vi "AnalysisData2.vi"() -> ()   [LabVIEW 2011]
panel:
  out "RunningIndexStart 2":dbl
  out "RunningIndexStart":dbl
  out "子数组":string[](array[string])
  out "EXCEL读取":string[][](array[string])
  in  "路径":path
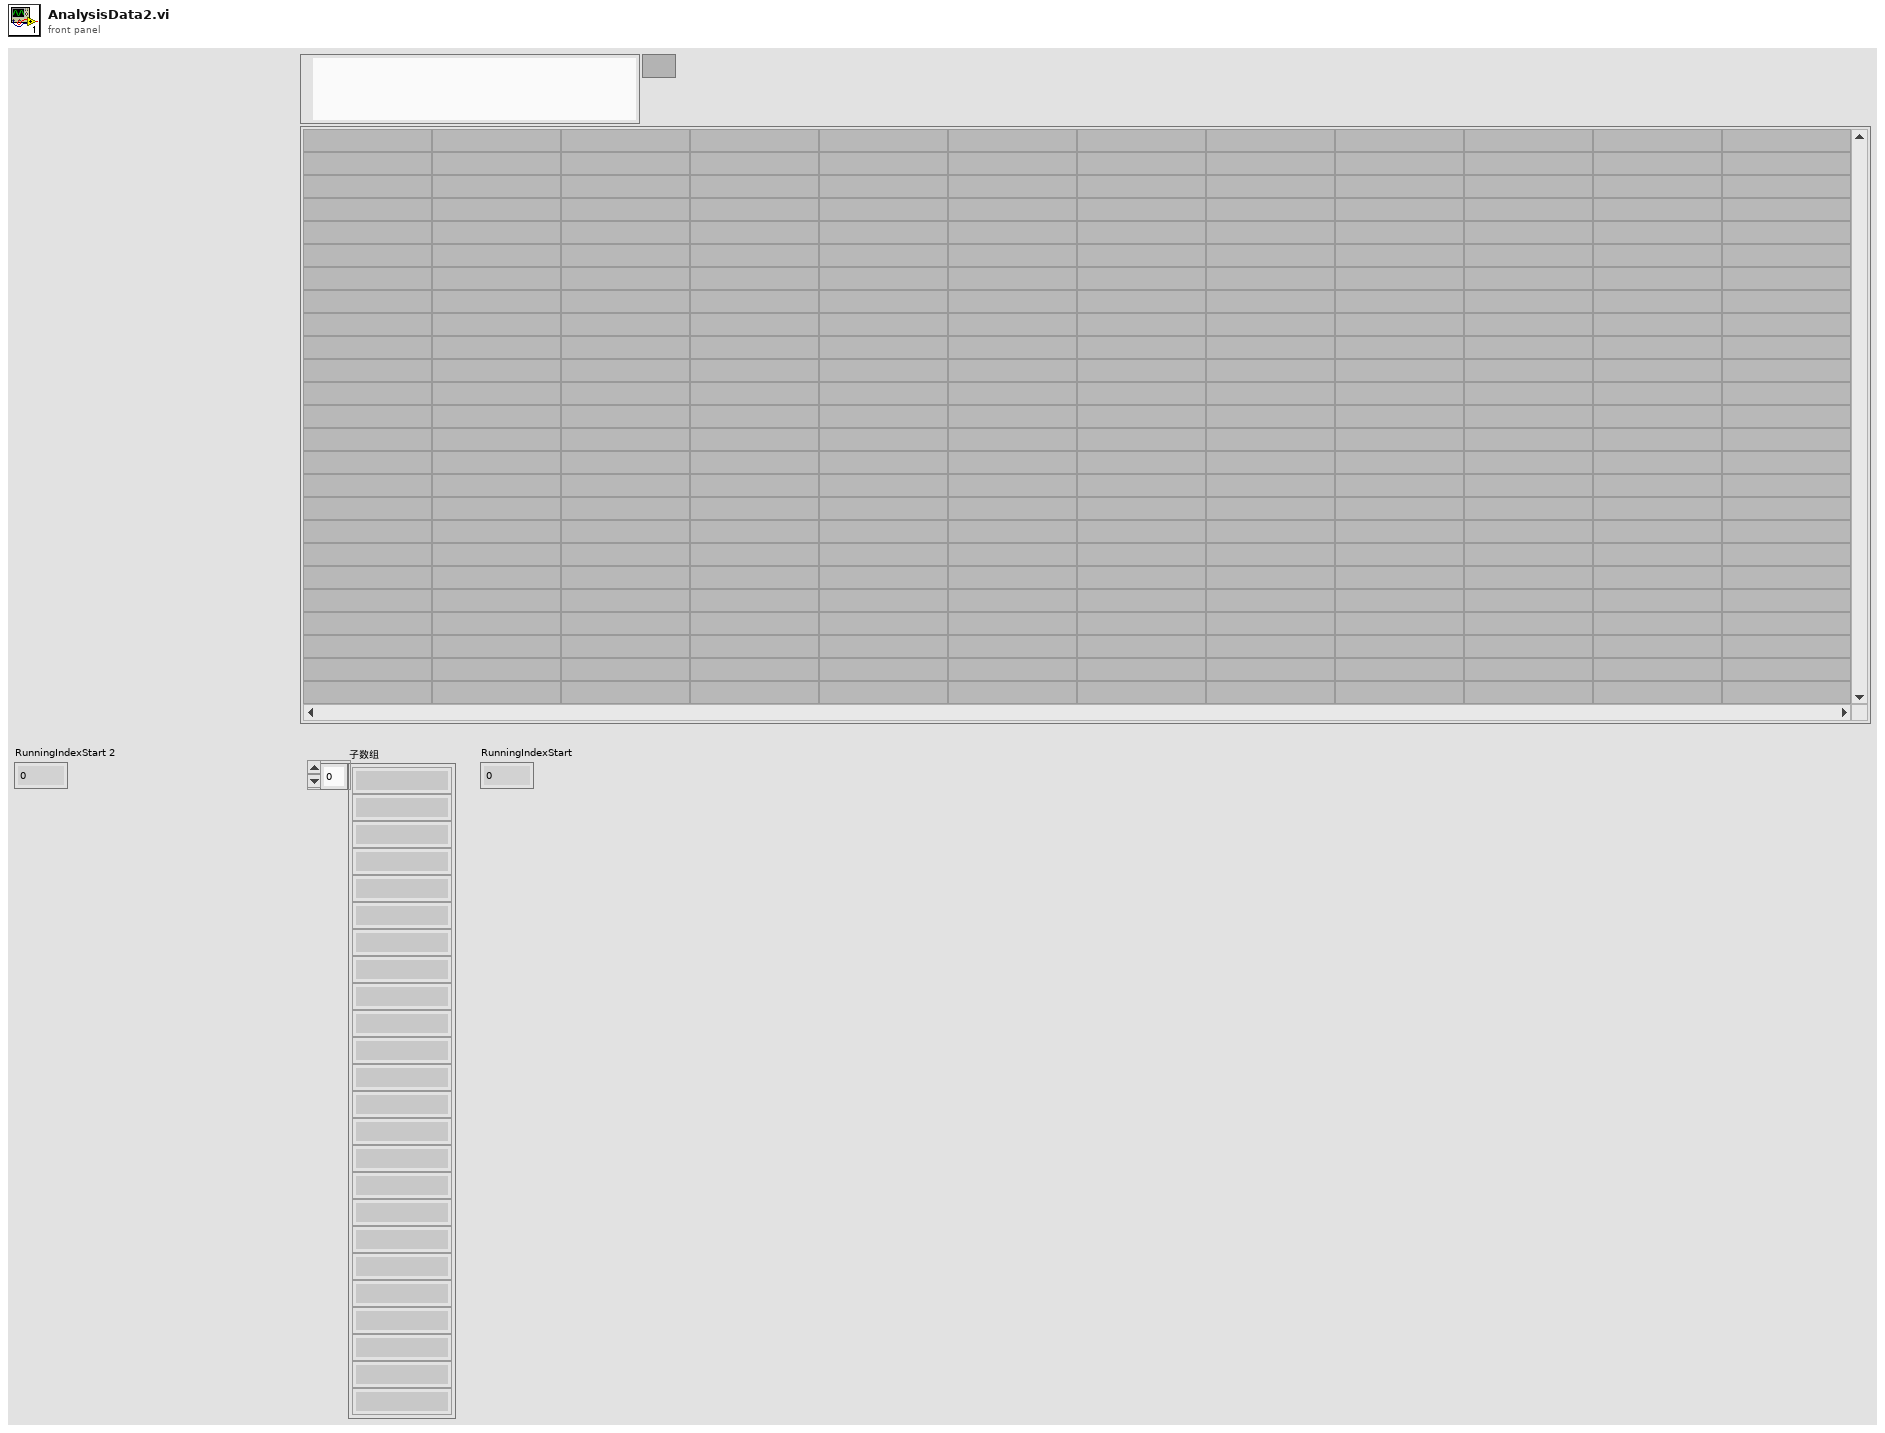
[diagram p1: front panel]
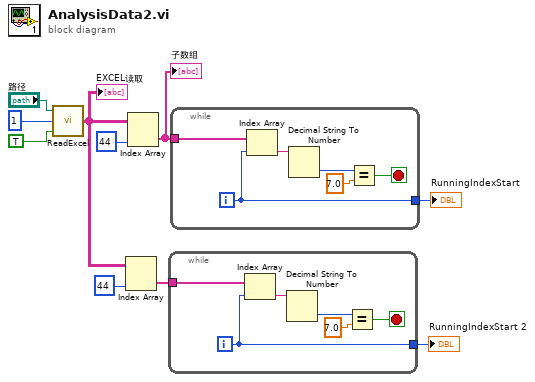
[diagram p0: block diagram]
diagram:
  n1 = call "ReadExcel.vi"("读出文本"=TRUE, "导出sheet位号"=i8 1, "路径"="路径") -> ("EXCEL读取"=w1:string[][])
  "EXCEL读取" <- w1
  n2 = Index Array(array=w1, index (col)=44 ("禁用的索引 (列)")) -> (element=w3:string[])  [unwired: 1 in]
  n3 = Index Array(array=w1, index (col)=44 ("禁用的索引 (列)")) -> (element=w6:string[])  [unwired: 1 in]
  "子数组" <- w6
  n4 = while {
    tunnel: w3 -> [w16]
    tunnel: [w11] -> w2
    i -> [w11]
    stop <- w12 stop-if-true
    n5 = Index Array(array=w16, index=w11) -> (element=w14:string)
    n6 = Decimal String To Number(string=w14) -> (number=w13:i32)  [unwired: 2 in, 1 out]
    n7 = Equal?(x=w13, y=7.0) -> (x = y?=w12:bool)
  }
  "RunningIndexStart 2" <- w2
  n8 = while {
    tunnel: w6 -> [w22]
    tunnel: [w17] -> w5
    i -> [w17]
    stop <- w18 stop-if-true
    n9 = Index Array(array=w22, index=w17) -> (element=w20:string)
    n10 = Decimal String To Number(string=w20) -> (number=w19:i32)  [unwired: 2 in, 1 out]
    n11 = Equal?(x=w19, y=7.0) -> (x = y?=w18:bool)
  }
  "RunningIndexStart" <- w5
